vi "RT_Lissajou_fit.vi"() -> ()   [LabVIEW 2019]
uses:
  <vilib>/Platform/TimedLoop/XDataNode/timing_clust.ctl
  <vilib>/Platform/TimedLoop/XDataNode/nitl_modes.ctl
  <vilib>/Platform/TimedLoop/XDataNode/wakeup.ctl
  <vilib>/FPGAPlugInAG/myRIO-1900/niLvFpga_Open_myRIO-1900.vi
  <vilib>/rvi/interface/common/dynamic/niFpgaDynamicAddResources.vi
  <vilib>/Utility/error.llb/Error Cluster From Error Code.vi
  <vilib>/rvi/errors/niLvFpgaAdjustHostInterfaceError.vi
  <vilib>/gmath/NumericalOptimization/Nonlinear Curve Fit LM.vi
  <vilib>/platform/TimedLoop/XDataNode/XDataNode.xnode
  <vilib>/rvi/interface/nirviOpenFPGA/nirviOpenFPGA.xnode
  FPGA Bitfiles/studentchallenge_FPGATarget_FPGA1RADC1WDAC2A_R8uuw9uWLNg.lvbitx
  <vilib>/rvi/interface/nirviReadWriteControl/nirviReadWriteControl.xnode
  <vilib>/Platform/TimedLoop/XDataNode/XDNodeRunTimeDep.lvlib
  <vilib>/gmath/NI_Gmath.lvlib
  <vilib>/Analysis/NI_AALBase.lvlib
  NiFpgaLv.dll
  <vilib>/rvi/interface/Simulation/niFpgaSimulationCallBeginRW.vi
panel:
  in  "Loop time (us)":i64=2000
  out "Fit":cluster{"X":dbl[], "Y":dbl[]}[](graph)
  out "Fit parameters":dbl[](array[numeric])=[0.26052296362991306, 0.4846685346905812, 1.4414779367760795, 1.587951197219736, -0.41010589812925907]
  out "Lissajou":cluster{"X":dbl[], "Y":dbl[]}[](graph)=[{"X"=[1.226806640625, 1.248779296875, 1.28173828125, 1.31103515625, 1.336669921875, 1.3623046875, 1.38671875, 1.4111328125, 1.427001953125, 1.4501953125, 1.248779296875, 1.28173828125, 1.31103515625, 1.336669921875, 1.3623046875, 1.38671875, 1.4111328125, 1.427001953125, 1.4501953125, 1.475830078125, 1.28173828125, 1.31103515625, 1.336669921875, 1.3623046875, 1.38671875, 1.4111328125, 1.427001953125, 1.4501953125, 1.475830078125, 1.50390625, 1.31103515625, 1.336669921875, 1.3623046875, 1.38671875, 1.4111328125, 1.427001953125, 1.4501953125, 1.475830078125, 1.50390625, 1.52587890625, 1.336669921875, 1.3623046875, 1.38671875, 1.4111328125, 1.427001953125, 1.4501953125, 1.475830078125, 1.50390625, 1.52587890625, 1.55029296875, 1.3623046875, 1.38671875, 1.4111328125, 1.427001953125, 1.4501953125, 1.475830078125, 1.50390625, 1.52587890625, 1.55029296875, 1.568603515625, 1.38671875, 1.4111328125, 1.427001953125, 1.4501953125, 1.475830078125, 1.50390625, 1.52587890625, 1.55029296875, 1.568603515625, 1.578369140625, 1.4111328125, 1.427001953125, 1.4501953125, 1.475830078125, 1.50390625, 1.52587890625, 1.55029296875, 1.568603515625, 1.578369140625, 1.58447265625], "Y"=[1.99951171875, 2.032470703125, 2.05810546875, 2.071533203125, 2.07763671875, 2.076416015625, 2.0703125, 2.0556640625, 2.04345703125, 2.025146484375, 2.032470703125, 2.05810546875, 2.071533203125, 2.07763671875, 2.076416015625, 2.0703125, 2.0556640625, 2.04345703125, 2.025146484375, 2.003173828125, 2.05810546875, 2.071533203125, 2.07763671875, 2.076416015625, 2.0703125, 2.0556640625, 2.04345703125, 2.025146484375, 2.003173828125, 1.968994140625, 2.071533203125, 2.07763671875, 2.076416015625, 2.0703125, 2.0556640625, 2.04345703125, 2.025146484375, 2.003173828125, 1.968994140625, 1.94091796875, 2.07763671875, 2.076416015625, 2.0703125, 2.0556640625, 2.04345703125, 2.025146484375, 2.003173828125, 1.968994140625, 1.94091796875, 1.9091796875, 2.076416015625, 2.0703125, 2.0556640625, 2.04345703125, 2.025146484375, 2.003173828125, 1.968994140625, 1.94091796875, 1.9091796875, 1.888427734375, 2.0703125, 2.0556640625, 2.04345703125, 2.025146484375, 2.003173828125, 1.968994140625, 1.94091796875, 1.9091796875, 1.888427734375, 1.865234375, 2.0556640625, 2.04345703125, 2.025146484375, 2.003173828125, 1.968994140625, 1.94091796875, 1.9091796875, 1.888427734375, 1.865234375, 1.854248046875]}]
  in  "stop":bool
  out "?":dbl(graph)=1.58447265625
  out "Finished Late? [i-1]":bool
  out "?":dbl(graph)=1.854248046875
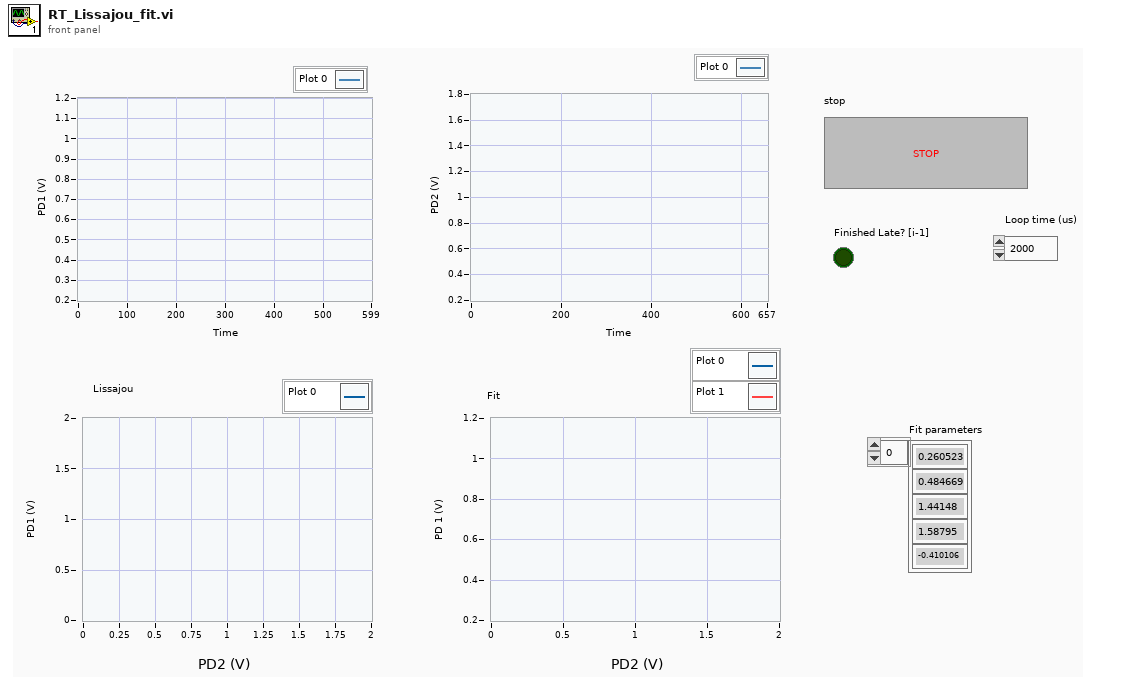
[diagram p1: front panel]
types:
  T1 = typedef "XDNodeRunTimeDep.lvlib/timing_clust.ctl" = cluster{"Expected End [f-1]":u64, "Actual End [f-1]":u64, "Finished Late? [f-1]":bool, "Expected End [i-1]":u64, "Actual End [i-1]":u64, "Finished Late? [i-1]":bool, "Expected Start [i]":u64, "Actual Start [i]":u64, "Expected Start [f]":u64, "Actual Start [f]":u64, "Source Name":string, "Structure Name":string, "Period":i64, "Deadline":i64, "Offset":i64, "Start":i64, "Priority":i32, "Timeout":i32, "Mode":T2, "Wakeup Reason":T3, "Error":errorcluster, "Source Type":string, "Secondary Source Type":string, "Global End Time":u64, "Global Start Time":u64, "Frame Duration":u64, "Iteration Duration":u64, "Assigned CPU":i32, "I/O Scan Engine Mode":u32}
  T2 = typedef "XDNodeRunTimeDep.lvlib/nitl_modes.ctl" = enum32{"No Change", "Process missed periods, maintain original phase", "Discard missed periods, maintain original phase", "Process missed periods, ignore original phase", "Discard missed periods, ignore original phase"}
  T3 = typedef "XDNodeRunTimeDep.lvlib/wakeup.ctl" = enum32{"Normal", "Aborted", "Asynchronous wakeup", "Timing source error", "Timed loop error", "Timeout"}
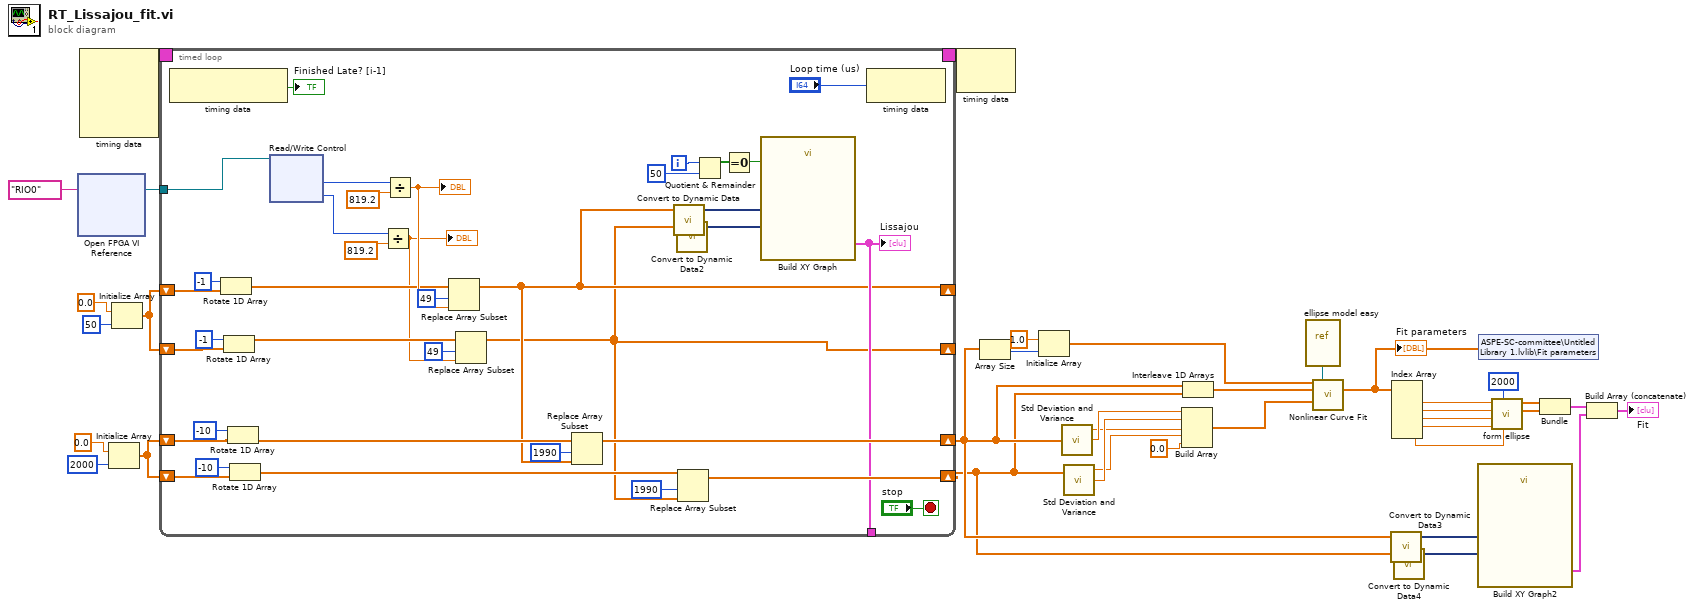
[diagram p0: block diagram]
diagram:
  n1 = xnode "Open FPGA VI Reference"("resource name"=tag "RIO0") -> ("FPGA VI Reference Out"=w34:refnum<k20>)  [unwired: 1 in, 1 out]
  n2 = node-c288() -> (w37:T1)  [unwired: 4 in]
  n3 = Initialize Array(0.0 ("element"), 2000 ("dimension size")) -> (w7:dbl[])
  n4 = Initialize Array(0.0 ("element"), 50 ("dimension size")) -> (w8:dbl[])
  n5 = timed-loop {
    timing: w37 -> [_]
    timing-out: [_] -> w36
    tunnel: w34 -> [w68]
    shift-right: [w39] -> _
    shift-left: w8 -> [w46]
    shift-right: [w40] -> _
    shift-left: w8 -> [w47]
    shift-right: [w45] -> w2
    shift-left: w7 -> [w44]
    shift-right: [w43] -> w3
    shift-left: w7 -> [w42]
    tunnel: [w41] -> _
    i -> [w65]
    stop <- "stop" stop-if-true
    n6 = node-c288() -> (→"Finished Late? [i-1]":bool)  [unwired: 1 in]
    n7 = Rotate 1D Array(1:w47, 2:-1 ("n")) -> (0:w50:dbl[])
    n8 = Rotate 1D Array(1:w46, 2:-1 ("n")) -> (0:w49:dbl[])
    n9 = Rotate 1D Array(1:w42, 2:-10 ("n")) -> (0:w54:dbl[])
    n10 = Rotate 1D Array(1:w44, 2:-10 ("n")) -> (0:w55:dbl[])
    n11 = xnode "Read/Write Control"("FPGA VI Reference In"=w68) -> ("PD1"=w73:u16, "PD2"=w70:u16)  [unwired: 1 in, 2 out]
    n12 = Divide(x=w70, y=819.2) -> (x/y=w48:dbl)
    "?" <- w48
    n13 = Divide(x=w73, y=819.2) -> (x/y=w51:dbl)
    "?" <- w51
    n14 = Replace Array Subset(array=w50, new element=w51, index=49) -> (w40:dbl[])
    n15 = Replace Array Subset(array=w49, new element=w48, index=49) -> (w39:dbl[])
    n16 = Replace Array Subset(array=w54, new element=w40, index=1990) -> (w43:dbl[])
    n17 = call "Convert to Dynamic Data"("Array"=w40) -> ("Dynamic Data Type"=w67:dynamicdata)  [unwired: 3 in]
    n18 = call "Convert to Dynamic Data2"("Array"=w39) -> ("Dynamic Data Type"=w66:dynamicdata)  [unwired: 3 in]
    n19 = Replace Array Subset(array=w55, new element=w39, index=1990) -> (w45:dbl[])
    n20 = Quotient & Remainder(x=w65, y=50) -> (x-y*floor(x/y)=w62:i32)  [unwired: 1 out]
    n21 = Equal To 0?(x=w62) -> (x = 0?=w63:bool)
    n22 = call "Build XY Graph"("Reset"=w63, "Y Input"=w66, "X Input"=w67) -> ("XY Graph"=w41:cluster{"X":dbl[], "Y":dbl[]}[])  [unwired: 7 in, 1 out]
    "Lissajou" <- w41
    n23 = node-c288("Loop time (us)") -> ()  [unwired: 1 out]
  }
  n24 = node-c288(w36) -> ()  [unwired: 1 out]
  n25 = Array Size(array=w3) -> (size(s)=w33:i32)
  n26 = Initialize Array(1.0 ("element"), w33) -> (w30:dbl[])
  n27 = call <vilib>:"Std Deviation and Variance.vi"("X"=w3) -> ("mean"=w14:dbl, "standard deviation"=w16:dbl)  [unwired: 1 in, 1 out]
  n28 = call <vilib>:"Std Deviation and Variance.vi"("X"=w2) -> ("mean"=w13:dbl, "standard deviation"=w15:dbl)  [unwired: 1 in, 1 out]
  n29 = Build Array(w16, w15, w14, w13, 0.0 ("element")) -> (w17:dbl[])
  n30 = Interleave 1D Arrays(w3, w2) -> (w29:dbl[])
  n31 = vi-ref "ellipse model easy.vi"() -> (w31:refnum<vi>)
  n32 = call-poly <vilib>:"Nonlinear Curve Fit.vi"("Y"=w30, "f(x,a)"=w31, "X"=w29, "initial parameters"=w17) -> ("best fit parameters"=w19:dbl[])  [unwired: 6 in, 5 out]
  "Fit parameters" <- w19
  n33 = call "Convert to Dynamic Data3"("Array"=w3) -> ("Dynamic Data Type"=w5:dynamicdata)  [unwired: 3 in]
  n34 = Index Array(array=w19) -> (element #1=w28:dbl, element #2=w27:dbl, element #3=w26:dbl, element #4=w25:dbl, element #5=w20:dbl)  [unwired: 5 in]
  n35 = call "Convert to Dynamic Data4"("Array"=w2) -> ("Dynamic Data Type"=w4:dynamicdata)  [unwired: 3 in]
  n36 = call "Build XY Graph2"("Y Input"=w4, "X Input"=w5) -> ("XY Graph"=w1:cluster{"X":dbl[], "Y":dbl[]}[])  [unwired: 8 in, 1 out]
  n37 = shared-variable "ASPE-SC-committee\\Untitled Library 1.lvlib\\Fit parameters"(w19) -> ()  [unwired: 1 in, 1 out]
  n38 = call "form ellipse.vi"("alpha"=w20, "samples"=2000, "y0"=w25, "x0"=w26, "b"=w27, "a"=w28) -> ("Y"=w21:dbl[], "X"=w22:dbl[])  [unwired: 4 in]
  n39 = Bundle("X"=w22, "Y"=w21) -> (w23:cluster{"X":dbl[], "Y":dbl[]})  [unwired: 1 in]
  n40 = Build Array (concatenate)(w23, w1) -> (→"Fit":cluster{"X":dbl[], "Y":dbl[]}[])
